vi "ProjectProviderLinker.vi"(11 "Required input":bool) -> ()   [LabVIEW 2019]
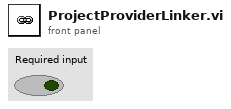
[diagram p1: front panel]
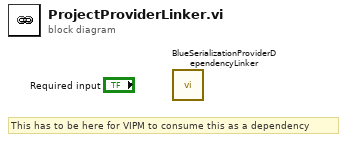
[diagram p0: block diagram]
diagram:
  # "This has to be here for VIPM to consume this as a dependency"
  n1 = call <resource>:"BlueSerializationProviderDependencyLinker.vi"() -> ()  [unwired: 12 in]
